vi "Round Position (uSMC).vi"(8 "error in":errorcluster, 9 "Step":u8(slide) scale=0.0..3.0, 10 "index":i32, 11 "Position(value)":dbl) -> (0 "error out":errorcluster, 3 "Position(rounded)":dbl)   [LabVIEW 2010, in "SignalWriterMH110203USBStepperMotor.lvclass"]
uses:
  SignalWriterMH110203USBStepperMotor.lvclass
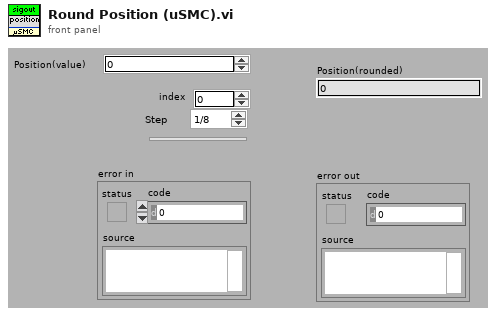
[diagram p1: front panel]
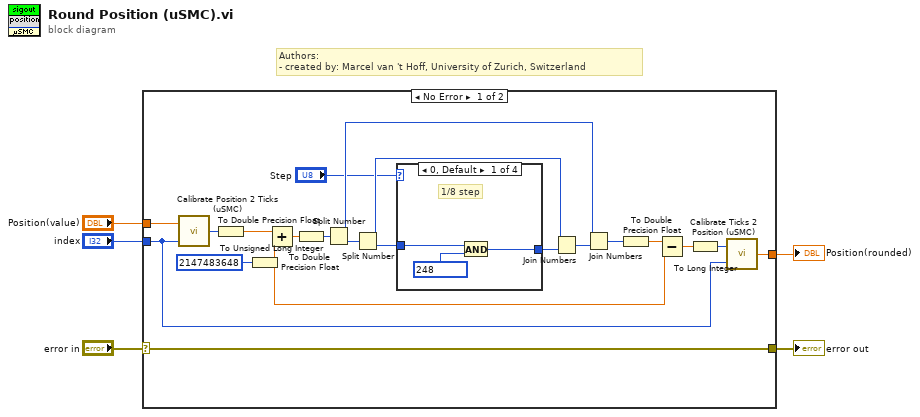
[diagram p0: block diagram]
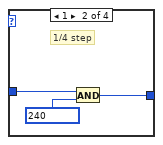
[diagram p2: hidden frame]
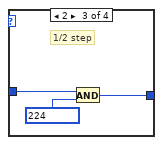
[diagram p3: hidden frame]
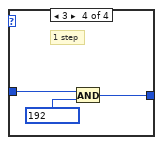
[diagram p4: hidden frame]
diagram:
  # "Authors: \n- created by: Marcel van 't Hoff, University of Zurich, Switzerland"
  n1 = case shown="No Error" "error in" {
    selector: "error in" -> [w6 w39]
    tunnel: [w26 _] -> w5
    tunnel: "Position(value)" -> [w25 _]
    tunnel: "index" -> [w16 _]
    tunnel: [w6 w39] -> w1
    frame No Error {
      n2 = call "Calibrate Position 2 Ticks (uSMC).vi"("array index"=w16, "value"=w25) -> ("value ticks"=w24:i32)
      n3 = To Double Precision Float(number=w24) -> (double precision float=w13:dbl)
      n4 = To Double Precision Float(number=u32 2147483648 ("value ticks")) -> (double precision float=w9:dbl)
      n5 = Add(x=w13, y=w9) -> (x+y=w15:dbl)
      n6 = To Unsigned Long Integer(number=w15) -> (unsigned 32bit integer=w12:u32)
      n7 = Split Number(x=w12) -> (hi(x)=w19:u16, lo(x)=w23:u16)
      n8 = Split Number(x=w23) -> (hi(x)=w18:u8, lo(x)=w22:u8)
      n9 = case shown="0, Default" "Step" {
        tunnel: w22 -> [w29 w32 w35 w38]
        tunnel: [w27 w30 w33 w36] -> w21
        frame 0, Default {
          # "1/8 step"
          n10 = And(x=w29, y=u8 248) -> (x .and. y?=w27:u8)
        }
        frame 1 {
          # "1/4 step"
          n11 = And(x=w32, y=u8 240) -> (x .and. y?=w30:u8)
        }
        frame 2 {
          # "1/2 step"
          n12 = And(x=w35, y=u8 224) -> (x .and. y?=w33:u8)
        }
        frame 3 {
          # "1 step"
          n13 = And(x=w38, y=u8 192) -> (x .and. y?=w36:u8)
        }
      }
      n14 = Join Numbers(hi=w18, lo=w21) -> ((hi.lo)=w20:u16)
      n15 = Join Numbers(hi=w19, lo=w20) -> ((hi.lo)=w17:u32)
      n16 = To Double Precision Float(number=w17) -> (double precision float=w11:dbl)
      n17 = Subtract(x=w11, y=w9) -> (x-y=w10:dbl)
      n18 = To Long Integer(number=w10) -> (32bit integer=w8:i32)
      n19 = call "Calibrate Ticks 2 Position (uSMC).vi"("array index"=w16, "ticks"=w8) -> ("value"=w26:dbl)
    }
    frame Error {
    }
  }
  "Position(rounded)" <- w5
  "error out" <- w1
